vi "DMM Settings Dialog.vi"(11 "DMM Parameters":T1[](array[typedef]) {"Resolution in Digits" items=["3 1/2"=3.5, "4 1/2"=4.5, "5 1/2"=5.5, "6 1/2"=6.5, "7 1/2"=7.5]}) -> (3 "DMM Parameters out":T1[](array[typedef]) caption="DMM Parameters" {"Resolution in Digits" items=["3 1/2"=3.5, "4 1/2"=4.5, "5 1/2"=5.5, "6 1/2"=6.5, "7 1/2"=7.5]})   [LabVIEW 2021, in "PMIC Common.lvlib"]
uses:
  PMIC Common.lvlib
  controls/UI DMM Parameters.ctl
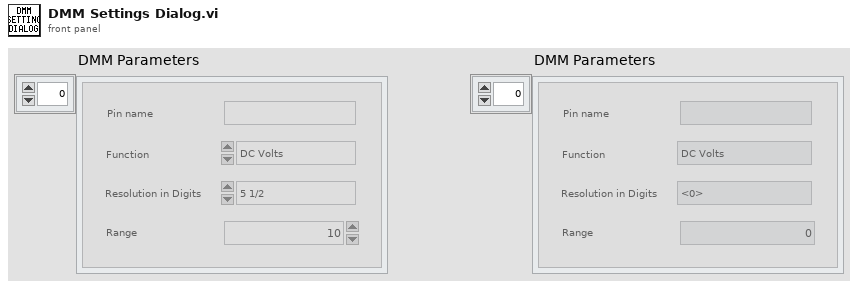
[diagram p1: front panel]
types:
  T1 = typedef "PMIC Common.lvlib/UI DMM Parameters.ctl" = cluster{"Pin name":string, "Function":enum16{"DC Volts", "AC Volts", "DC Current", "AC Current", "2-wire Resistance", "4-wire Resistance", "Diode", "Frequency", "Period", "AC Volts DC Coupled", "Capacitance", "Inductance", "Temperature"}, "Resolution in Digits":dbl, "Range":dbl}
  T2 = enum32{"Invalid", "Standard", "Closed", "Hidden", "Minimized", "Maximized"}
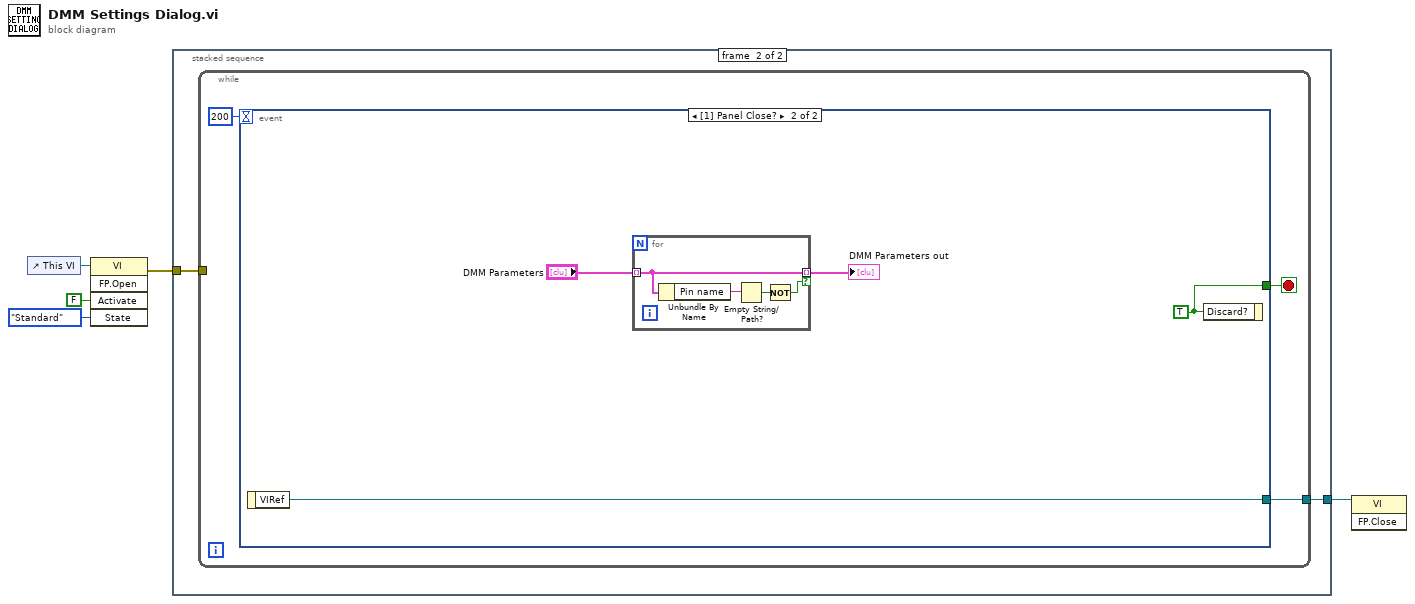
[diagram p0: block diagram]
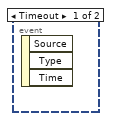
[diagram p3: hidden frame]
diagram:
  n1 = control-ref of="This VI"() -> (w5:refnum<vi>)
  n2 = invoke class="VI" method="FP.Open"(reference=w5, "Activate"=FALSE ("Activate?"), "State"=T2."Standard") -> (error out=w2:errorcluster)  [unwired: 2 in, 4 out]
  n3 = stacked-sequence {
    tunnel: w2 -> [_ w7]
    tunnel: [_ w6] -> w1
    frame #0 {
    }
    frame #1 {
      n4 = while {
        tunnel: [w8] -> w6
        tunnel: w7 -> [_]
        stop <- w10 stop-if-true
        n5 = event shown="[1] Panel Close?" {
          selector: _ -> [_ _]
          dyn-events: _ -> [_ _]
          timeout: 200 -> [_ _]
          tunnel: [_ w13] -> w10
          tunnel: [_ w14] -> w8
          event Timeout {
            n6 = event-data() -> ()  [unwired: 1 in, 3 out]
          }
          event Panel Close? {
            w13 = TRUE ("Discard?")
            n7 = event-data() -> ("VIRef"=w14:refnum<vi>)  [unwired: 1 in]
            n8 = for {
              tunnel: "DMM Parameters" -> [w16] mode=indexing
              tunnel: [w16] -> w11 mode=indexing if=w15
              n9 = Unbundle By Name(w16) -> ("Pin name"=w18:string)
              n10 = Empty String/Path?(string/path=w18) -> (empty?=w17:bool)
              n11 = Not(x=w17) -> (.not. x?=w15:bool)
            }
            "DMM Parameters out" <- w11
            n12 = event-data("Discard?"=w13) -> ()  [unwired: 1 in, 1 out]
          }
        }
      }
    }
  }
  n13 = invoke class="VI" method="FP.Close"(reference=w1) -> ()  [unwired: 2 in, 3 out]
